vi "calibrationElectrometer_logEvent_IntensityReq.vi"(8 "error in (no error)":errorcluster, 11 "logevent_IntensityReq_Ctl":T1={"calibrationElectrometerID"=0, "electId"=0, "intensity[1000]"=array[1000 elements], "masureTimestamp[2]"=[0.0, 0.0], "mode"=0, "packetId"=0, "size"=0, "temperature[2]"=[0.0, 0.0], "unit"="", "priority"=0}) -> (0 "error out":errorcluster, 2 "function return":i32, 3 "logevent_IntensityReq_Ctl out":T1)   [LabVIEW 2016, in "SALLV_calibrationElectrometer.lvlib"]
doc: "int calibrationElectrometer_shm_logEvent_IntensityReqLV(calibrationElectrometer_logevent_IntensityReqLV *logevent_IntensityReq_Ctl );"
uses:
  SALLV_calibrationElectrometer.lvlib
  DataTypes/logevent_IntensityReq.ctl
  SALLV_calibrationElectrometer.so
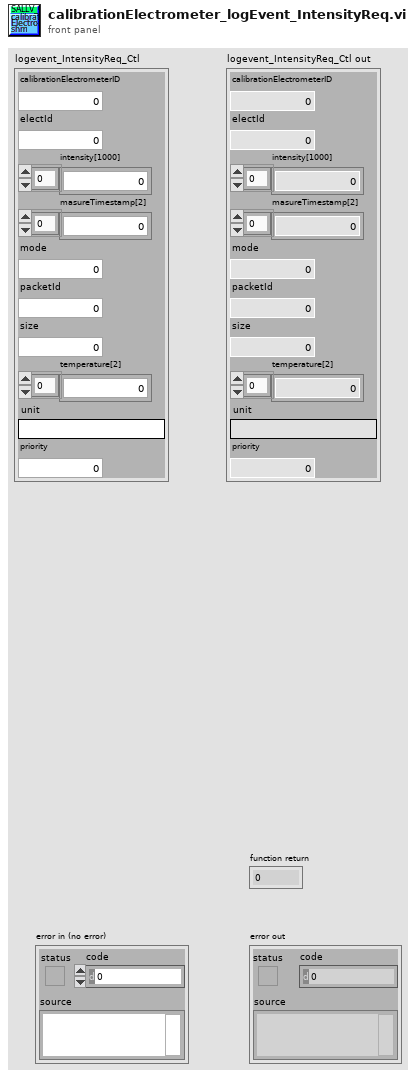
[diagram p1: front panel]
types:
  T1 = typedef "SALLV_calibrationElectrometer.lvlib/logevent_IntensityReq.ctl" = cluster{"calibrationElectrometerID":i16, "electId":i16, "intensity[1000]":dbl[], "masureTimestamp[2]":dbl[], "mode":u16, "packetId":u16, "size":u16, "temperature[2]":sgl[], "unit":string, "priority":i32}
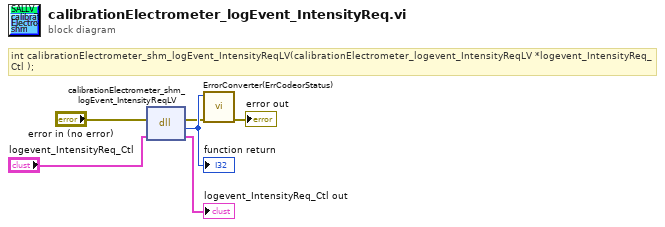
[diagram p0: block diagram]
diagram:
  # "int calibrationElectrometer_shm_logEvent_IntensityReqLV(calibrationElectrometer_logevent_IntensityReqLV *logevent_IntensityReq_Ctl );"
  n1 = dll-call lib="home/andres/Desktop/SAL_calibrationElectrometer/SALLV_calibrationElectrometer.*" fn="calibrationElectrometer_shm_logEvent_IntensityReqLV"(error in="error in (no error)", "logevent_IntensityReq_Ctl"="logevent_IntensityReq_Ctl") -> (error out=w2:errorcluster, w6:i32, "logevent_IntensityReq_Ctl"=→"logevent_IntensityReq_Ctl out":T1)  [unwired: 2 in, 1 out]
  "function return" <- w6
  n2 = call "ErrorConverter(ErrCodeorStatus).vi"("error in (no error)"=w2, "error code"=w6) -> ("error out"=→"error out":errorcluster)  [unwired: 9 in]
